vi "DecodeOurRobots.vi"(8 "error in":errorcluster, 9 "array":u8[](array[numeric]), 10 "Key":i32=5) -> (0 "error out":errorcluster, 1 "array w/ subset deleted out":u8[](array[numeric]), 3 "Our_Robots":T1(array[cluster]))   [LabVIEW 2017]
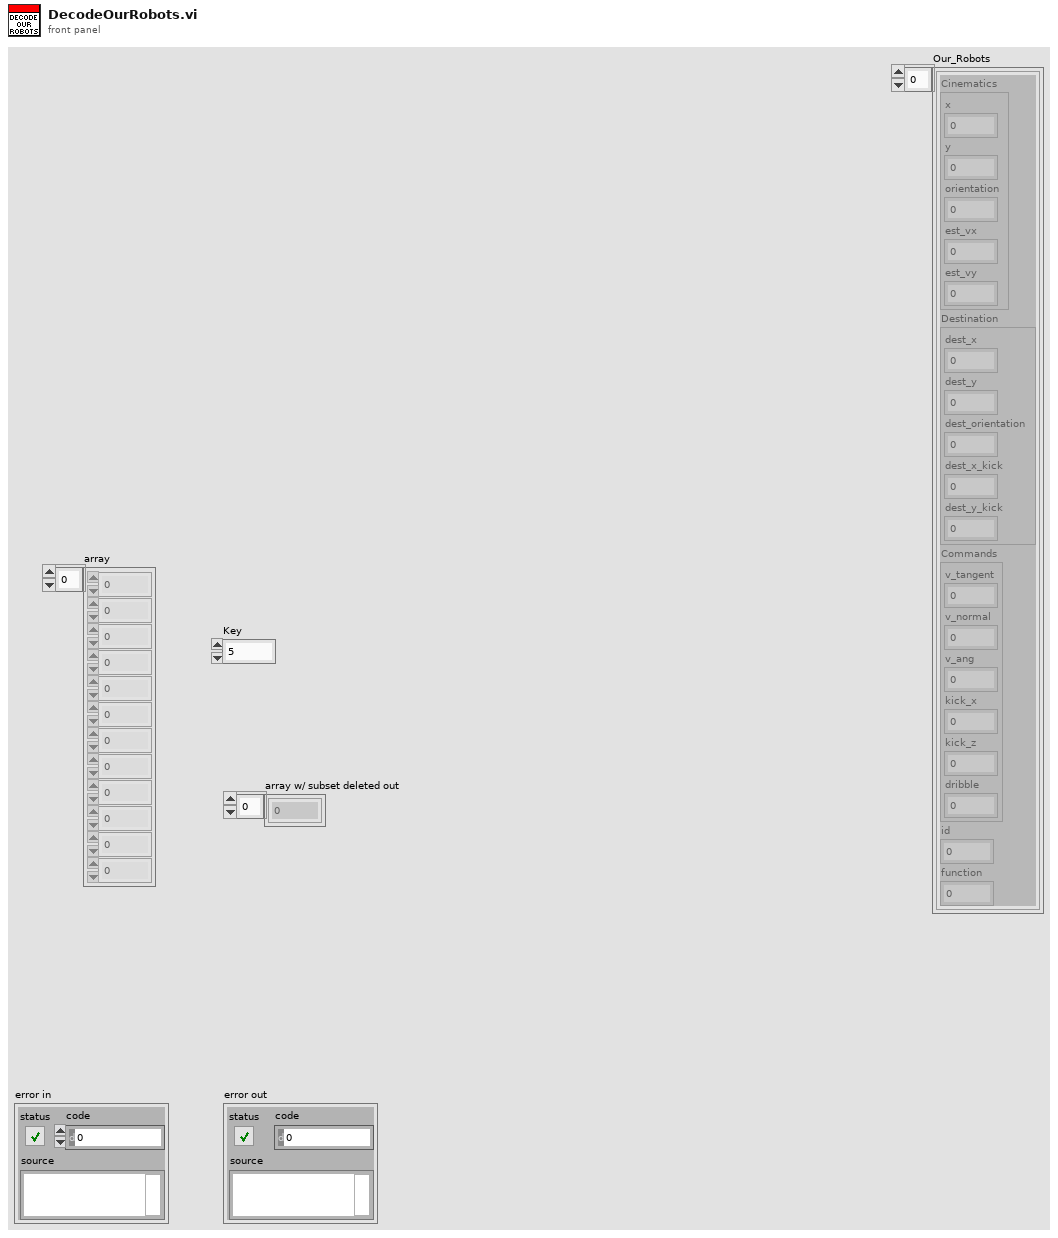
[diagram p1: front panel]
types:
  T1 = cluster{"Cinematics":cluster{"x":dbl, "y":dbl, "orientation":dbl, "est_vx":dbl, "est_vy":dbl}, "Destination":cluster{"dest_x":dbl, "dest_y":dbl, "dest_orientation":dbl, "dest_x_kick":dbl, "dest_y_kick":dbl}, "Commands":cluster{"v_tangent":dbl, "v_normal":dbl, "v_ang":dbl, "kick_x":dbl, "kick_z":dbl, "dribble":u32}, "id":u32, "function":u32}[]
  T2 = cluster{"Cinematics":cluster{"x":dbl, "y":dbl, "orientation":dbl, "est_vx":dbl, "est_vy":dbl}, "Destination":cluster{"dest_x":dbl, "dest_y":dbl, "dest_orientation":dbl, "dest_x_kick":dbl, "dest_y_kick":dbl}, "Commands":cluster{"v_tangent":dbl, "v_normal":dbl, "v_ang":dbl, "kick_x":dbl, "kick_z":dbl, "dribble":u32}, "id":u32, "function":u32}
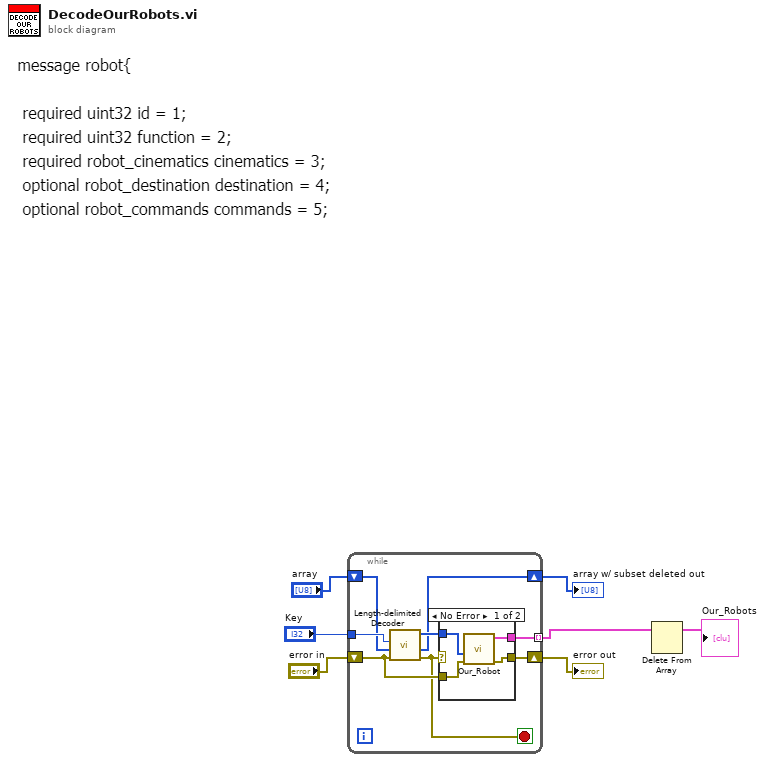
[diagram p0: block diagram]
diagram:
  n1 = while {
    tunnel: "Key" -> [w12]
    tunnel: [w10] -> w2 mode=indexing
    shift-right: [w13] -> w6
    shift-left: "error in" -> [w9]
    shift-right: [w14] -> w7
    shift-left: "array" -> [w11]
    stop <- w8 stop-if-true
    n2 = call "Length-delimited Decoder.vi"("error in (no error)"=w9, "Array"=w11, "Key"=w12) -> ("error out"=w8:errorcluster, "array w/ subset deleted"=w14:u8[], "Length-delimited"=w15:u8[])  [unwired: 5 in, 1 out]
    n3 = case shown="No Error" w8 {
      tunnel: [w17 w20] -> w13
      tunnel: w15 -> [w19 _]
      tunnel: w9 -> [w18 w20]
      tunnel: [w16 _] -> w10
      frame No Error {
        n4 = call "Our_Robot.vi"("error in"=w18, "Array"=w19) -> ("error out"=w17:errorcluster, "Our_Robots"=w16:T2)  [unwired: 7 in, 1 out]
      }
      frame Error {
      }
    }
  }
  "error out" <- w6
  "array w/ subset deleted out" <- w7
  n5 = Delete From Array(array=w2) -> (array with subset deleted=→"Our_Robots":T1)  [unwired: 2 in, 1 out]
